vi "BuildFilePath.vi"(1 "File Name":string="Sensors_DAQ1") -> (0 "Path":path=path "C:/Labview Test Data/2018-08-08/Sensors_DAQ1_Log.tdms")   [LabVIEW 2018]
uses:
  Global Variables.vi
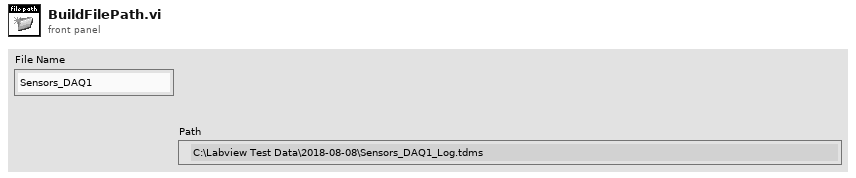
[diagram p1: front panel]
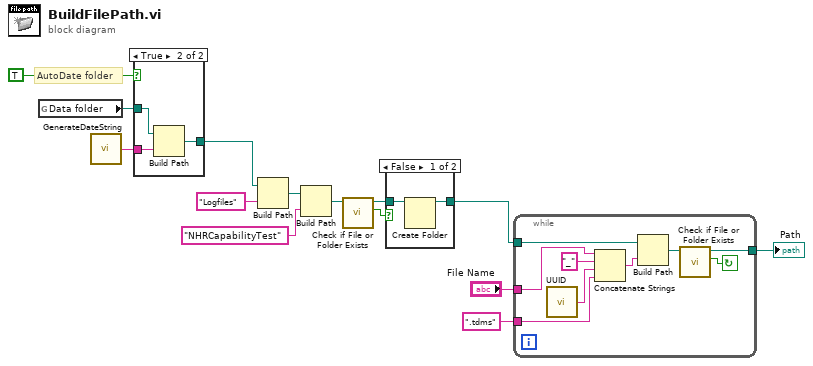
[diagram p0: block diagram]
diagram:
  # "AutoDate folder"
  n1 = global read "Global Variables.vi" "Data folder"() -> (w12:path)
  n2 = call "GenerateDateString.vi"() -> ("String"=w14:string)
  n3 = case shown="True" TRUE ("Auto Date folder") {
    tunnel: w12 -> [w15 w18]
    tunnel: [w15 w16] -> w7
    tunnel: w14 -> [_ w17]
    frame False {
    }
    frame True {
      n4 = Build Path(base path=w18, name or relative path=w17) -> (appended path=w16:path)
    }
  }
  n5 = Build Path(base path=w7, name or relative path="Logfiles") -> (appended path=w3:path)
  n6 = Build Path(base path=w3, name or relative path="NHRCapabilityTest") -> (appended path=w2:path)
  n7 = call <vilib>:"Check if File or Folder Exists.vi"("path"=w2) -> ("file or folder exists?"=w5:bool, "dup path"=w6:path)  [unwired: 8 in, 1 out]
  n8 = case shown="False" w5 {
    tunnel: w6 -> [w20 w21]
    tunnel: [w19 w21] -> w4
    frame False {
      n9 = Create Folder(path (use dialog)=w20) -> (created path=w19:path)  [unwired: 2 in, 2 out]
    }
    frame True {
    }
  }
  n10 = while {
    tunnel: "File Name" -> [w24]
    tunnel: ".tdms" ("Extension (.tdms)") -> [w26]
    tunnel: [w27] -> w9
    tunnel: w4 -> [w25]
    stop <- w29 continue-if-true
    n11 = call "UUID.vi"() -> ("UUID"=w22:string)
    n12 = Concatenate Strings(w24, "_" ("string"), w22, w26) -> (w28:string)
    n13 = Build Path(base path=w25, name or relative path=w28) -> (appended path=w30:path)
    n14 = call <vilib>:"Check if File or Folder Exists.vi"("path"=w30) -> ("file or folder exists?"=w29:bool, "dup path"=w27:path)  [unwired: 8 in, 1 out]
  }
  "Path" <- w9
